vi "Read Response.vi"(8 "error in (no error)":errorcluster, 11 "VISA resource name":refnum<visa-resource-name>) -> (0 "error out":errorcluster, 2 "Response":string, 3 "VISA resource name Out":refnum<visa-resource-name>, 5 "Buffer":string)   [LabVIEW 2024, in "CTIPicoVISA.lvlib"]
uses:
  CTIPicoVISA.lvlib
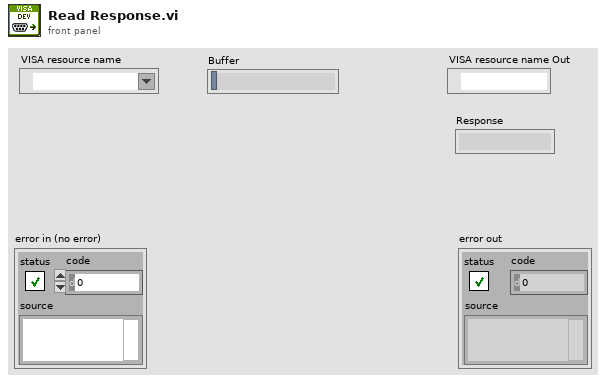
[diagram p1: front panel]
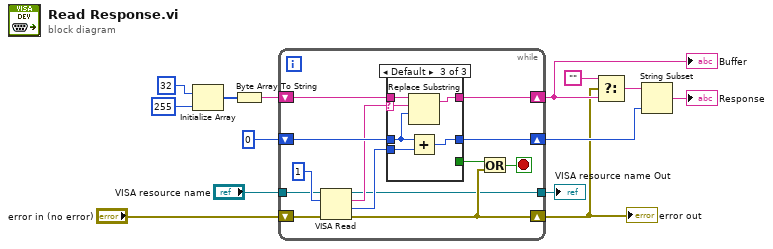
[diagram p0: block diagram]
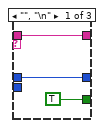
[diagram p2: hidden frame]
diagram:
  n1 = Initialize Array(u8 32 ("element"), 255 ("dimension size")) -> (w12:u8[])
  n2 = Byte Array To String(unsigned byte array=w12) -> (string=w8:string)
  n3 = while {
    shift-right: [w19] -> w2
    shift-left: "error in (no error)" -> [w27]
    shift-right: [w22] -> w4
    shift-left: w8 -> [w25]
    shift-right: [w23] -> w9
    shift-left: u32 0 -> [w24]
    tunnel: "VISA resource name" -> [w16]
    tunnel: [w15] -> w1
    stop <- w20 stop-if-true
    n4 = VISA Read(VISA resource name=w16, byte count=u32 1, error in (no error)=w27) -> (VISA resource name out=w15:refnum<visa-resource-name>, read buffer=w18:string, return count=w21:u32, error out=w19:errorcluster)
    n5 = case shown="Default" w18 {
      selector: w18 -> [_ _ w33]
      tunnel: w25 -> [w30 w32 w38]
      tunnel: w24 -> [w29 w31 w37]
      tunnel: [w29 w31 w36] -> w23
      tunnel: [w30 w32 w35] -> w22
      tunnel: w21 -> [_ _ w34]
      tunnel: [TRUE _ _] -> w17
      frame "", "\n" {
      }
      frame "\r" {
      }
      frame Default {
        n6 = Replace Substring(3:w37, 4:w33, 5:w38) -> (1:w35:string)  [unwired: 1 in, 1 out]
        n7 = Add(x=w37, y=w34) -> (x+y=w36:u32)
      }
    }
    n8 = Or(x=w17, y=w19) -> (x .or. y?=w20:bool)
  }
  "error out" <- w2
  "Buffer" <- w4
  "VISA resource name Out" <- w1
  n9 = Select(t="", s=w2, f=w4) -> (s? t:f=w10:string)
  n10 = String Subset(string=w10, length (rest)=w9) -> (substring=→"Response":string)  [unwired: 1 in]
